vi "CreateProxyDLL.vi"(8 "error in (no error)":errorcluster, 10 "Base Path":path, 11 "Web Service Importer in":refnum<k24>) -> (0 "error out":errorcluster, 1 "ErrorMessage":string, 2 "ErrorCode":i32(ring)=200 items=["kNoError"=200, "kUnknown"=201, "kUrlNotFoundOrBadWSDL"=202, "kBadlyFormattedURL"=203, "kBadHostname"=204], 3 "Web Service Importer out":refnum<k24>)   [LabVIEW 2017]
uses:
  e:/builds/penguin/labview/branches/2017/dev/dist/resource/WebServiceUtils.dll
  resource/WebServiceUtils.dll
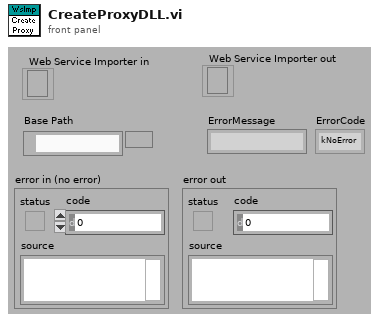
[diagram p1: front panel]
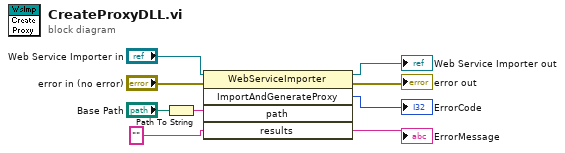
[diagram p0: block diagram]
diagram:
  n1 = Path To String(path="Base Path") -> (string=w5:string)
  n2 = invoke class="WebServiceImporter" method="ImportAndGenerateProxy"(reference="Web Service Importer in", error in="error in (no error)", "path"=w5, "results"="") -> (reference out=→"Web Service Importer out":refnum<k24>, error out=→"error out":errorcluster, "ImportAndGenerateProxy"=→"ErrorCode":i32, "results"=→"ErrorMessage":string)  [unwired: 1 in, 1 out]
